vi "_TestDemo.vi"() -> ()   [LabVIEW 2012]
panel:
  out "Motor speed":i32
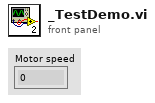
[diagram p1: front panel]
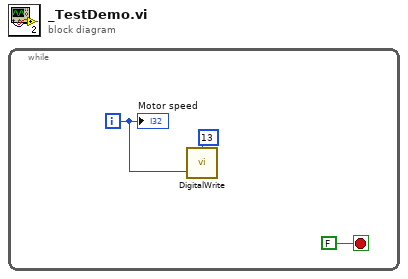
[diagram p0: block diagram]
diagram:
  n1 = while {
    i -> [w2]
    stop <- FALSE stop-if-true
    n2 = call "DigitalWrite.vi"("State"=w2, "Port"=u8 13) -> ()  [unwired: 1 in, 2 out]
    "Motor speed" <- w2
  }
